vi "Generate Permissions Integer.vi"(7 "Permissions":T1={"User Password"="", "Owner Password"="", "Printing"=enum."Allow Printing", "Allow Modify Contents"=FALSE, "Allow Copy"=FALSE, "Allow Modify Annotations"=TRUE, "Allow Fill In "=TRUE, "Allow Screen Readers"=FALSE, "Allow Assembly"=FALSE}, 11 "error in (no error)":errorcluster) -> (8 "Permissions":i32, 15 "error out":errorcluster)   [LabVIEW 2019, in "Exaprom PDF.lvlib"]
doc: "Version 1.0\nDeveloped by Jean-Marc Simard\nCopyright © 2011, Exaprom Inc.\nAll rights reserved.\nLicense: BSD\n\nWith iTextSharp 4.1.6 (http://itextsharp.sourceforge.net)\nunder Mozilla Public License Version 1.1\n(http://www.mozilla.org/MPL/MPL-1.1.html)"
uses:
  Controls/Initialization Controls/File Permission Parameters.ctl
  Exaprom PDF.lvlib
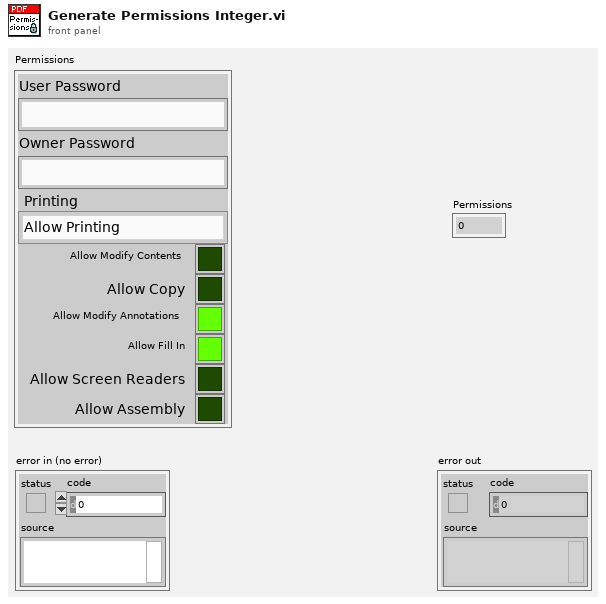
[diagram p1: front panel]
types:
  T1 = typedef "Exaprom PDF.lvlib/File Permission Parameters.ctl" = cluster{"User Password":string, "Owner Password":string, "Printing":enum16{"Allow Printing", "Allow Degraded Printing", "Don't Allow Printing"}, "Allow Modify Contents":bool, "Allow Copy":bool, "Allow Modify Annotations":bool, "Allow Fill In ":bool, "Allow Screen Readers":bool, "Allow Assembly":bool}
  T2 = enum16{"Allow Printing", "Allow Degraded Printing", "Don't Allow Printing"}
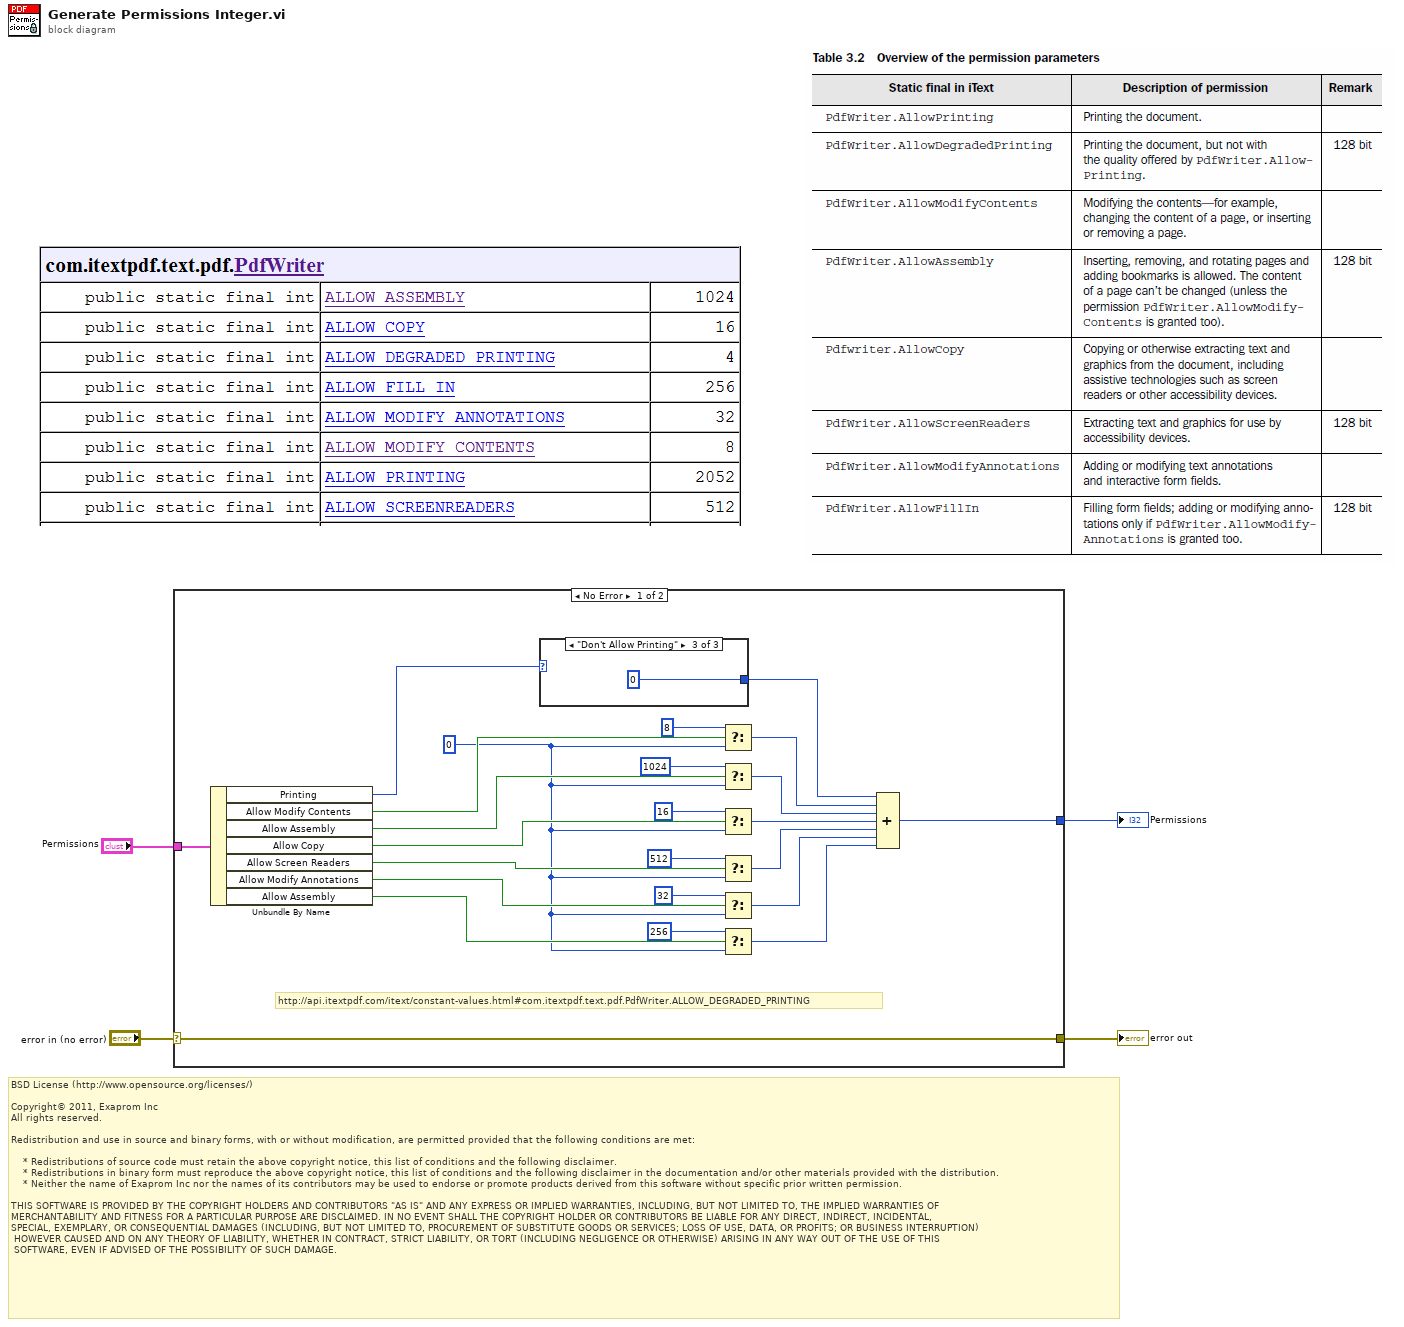
[diagram p0: block diagram]
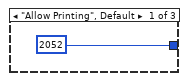
[diagram p2: hidden frame]
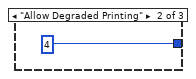
[diagram p3: hidden frame]
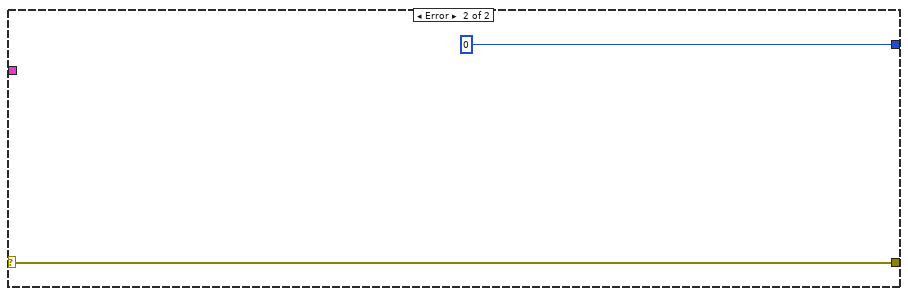
[diagram p4: hidden frame]
diagram:
  # "BSD License (http://www.opensource.org/licenses/)\n\nCopyright© 2011, Exaprom Inc\nAll rights reserved.\n\nRedistribution and use in source and binary forms, with or without modification, are permitted provided that the following conditions are met:\n\n    * Redistributions of source code must retain the above copyright notice, this list of conditions and the following disclaimer.\n    * Redistributions in binary form must reproduce the above copyright notice, this list of conditions and the following disclaimer in the documentation and/or other materials provided with the distribution.\n    * Neither the name of Exaprom Inc nor the names of its contributors may be used to endorse or promote products derived from this software without specific prior written permission.\n\nTHIS SOFTWARE IS PROVIDED BY THE COPYRIGHT HOLDERS AND CONTRIBUTORS \"AS IS\" AND ANY EXPRESS OR IMPLIED WARRANTIES, INCLUDING, BUT NOT LIMITED TO, THE IMPLIED WARRANTIES OF \nMERCHANTABILITY AND FITNESS FOR A PARTICULAR PURPOSE ARE DISCLAIMED. IN NO EVENT SHALL THE COPYRIGHT HOLDER OR CONTRIBUTORS BE LIABLE FOR ANY DIRECT, INDIRECT, INCIDENTAL,\nSPECIAL, EXEMPLARY, OR CONSEQUENTIAL DAMAGES (INCLUDING, BUT NOT LIMITED TO, PROCUREMENT OF SUBSTITUTE GOODS OR SERVICES; LOSS OF USE, DATA, OR PROFITS; OR BUSINESS INTERRUPTION)\n HOWEVER CAUSED AND ON ANY THEORY OF LIABILITY, WHETHER IN CONTRACT, STRICT LIABILITY, OR TORT (INCLUDING NEGLIGENCE OR OTHERWISE) ARISING IN ANY WAY OUT OF THE USE OF THIS\n SOFTWARE, EVEN IF ADVISED OF THE POSSIBILITY OF SUCH DAMAGE."
  n1 = case shown="No Error" "error in (no error)" {
    selector: "error in (no error)" -> [w28 w33]
    tunnel: [w28 w33] -> w4
    tunnel: "Permissions" -> [w27 _]
    tunnel: [w5 0] -> w1
    frame No Error {
      w15 = 0 ("permissions")
      # "http://api.itextpdf.com/itext/constant-values.html#com.itextpdf.text.pdf.PdfWriter.ALLOW_DEGRADED_PRINTING"
      n2 = Unbundle By Name(w27) -> ("Printing"=w26:T2, "Allow Modify Contents"=w25:bool, "Allow Assembly"=w23:bool, "Allow Copy"=w21:bool, "Allow Screen Readers"=w19:bool, "Allow Modify Annotations"=w17:bool, "Allow Assembly"=w16:bool)
      n3 = case shown="\"Don't Allow Printing\"" w26 {
        tunnel: [2052 ("permissions") 4 ("permissions") 0 ("permissions")] -> w12
        frame "Allow Printing", Default {
        }
        frame "Allow Degraded Printing" {
        }
        frame "Don't Allow Printing" {
        }
      }
      n4 = Select(t=8, s=w25, f=w15) -> (s? t:f=w11:i32)
      n5 = Select(t=1024, s=w23, f=w15) -> (s? t:f=w10:i32)
      n6 = Select(t=16, s=w21, f=w15) -> (s? t:f=w9:i32)
      n7 = Select(t=512, s=w19, f=w15) -> (s? t:f=w8:i32)
      n8 = Select(t=32, s=w17, f=w15) -> (s? t:f=w7:i32)
      n9 = Select(t=256, s=w16, f=w15) -> (s? t:f=w6:i32)
      n10 = Compound Arithmetic op=ADD(w12, w11, w10, w9, w8, w7, w6) -> (w5:i32)
    }
    frame Error {
    }
  }
  "error out" <- w4
  "Permissions" <- w1
